vi "Invert Data.vi"(8 "error in (no error)":errorcluster, 9 "Multiplot Representation In":T1, 10 "Actual Transform In":T5, 11 "3D Plot.lvclass in":refnum<class "3D Plot.lvclass">) -> (0 "error out":errorcluster, 1 "Multiplot Representation In":T1, 2 "Actual Transform Out":T5, 3 "3D Plot.lvclass out":refnum<class "3D Plot.lvclass">)   [LabVIEW 2020, in "3D Plot.lvclass"]
uses:
  3D Plot.lvclass
  Actual Transform.ctl
  Range Clusters.ctl
  Multiplot Representation.ctl
  Plot Representation.ctl
  Mesh Data.ctl
  3D Plot.lvclass/3D Plot.ctl
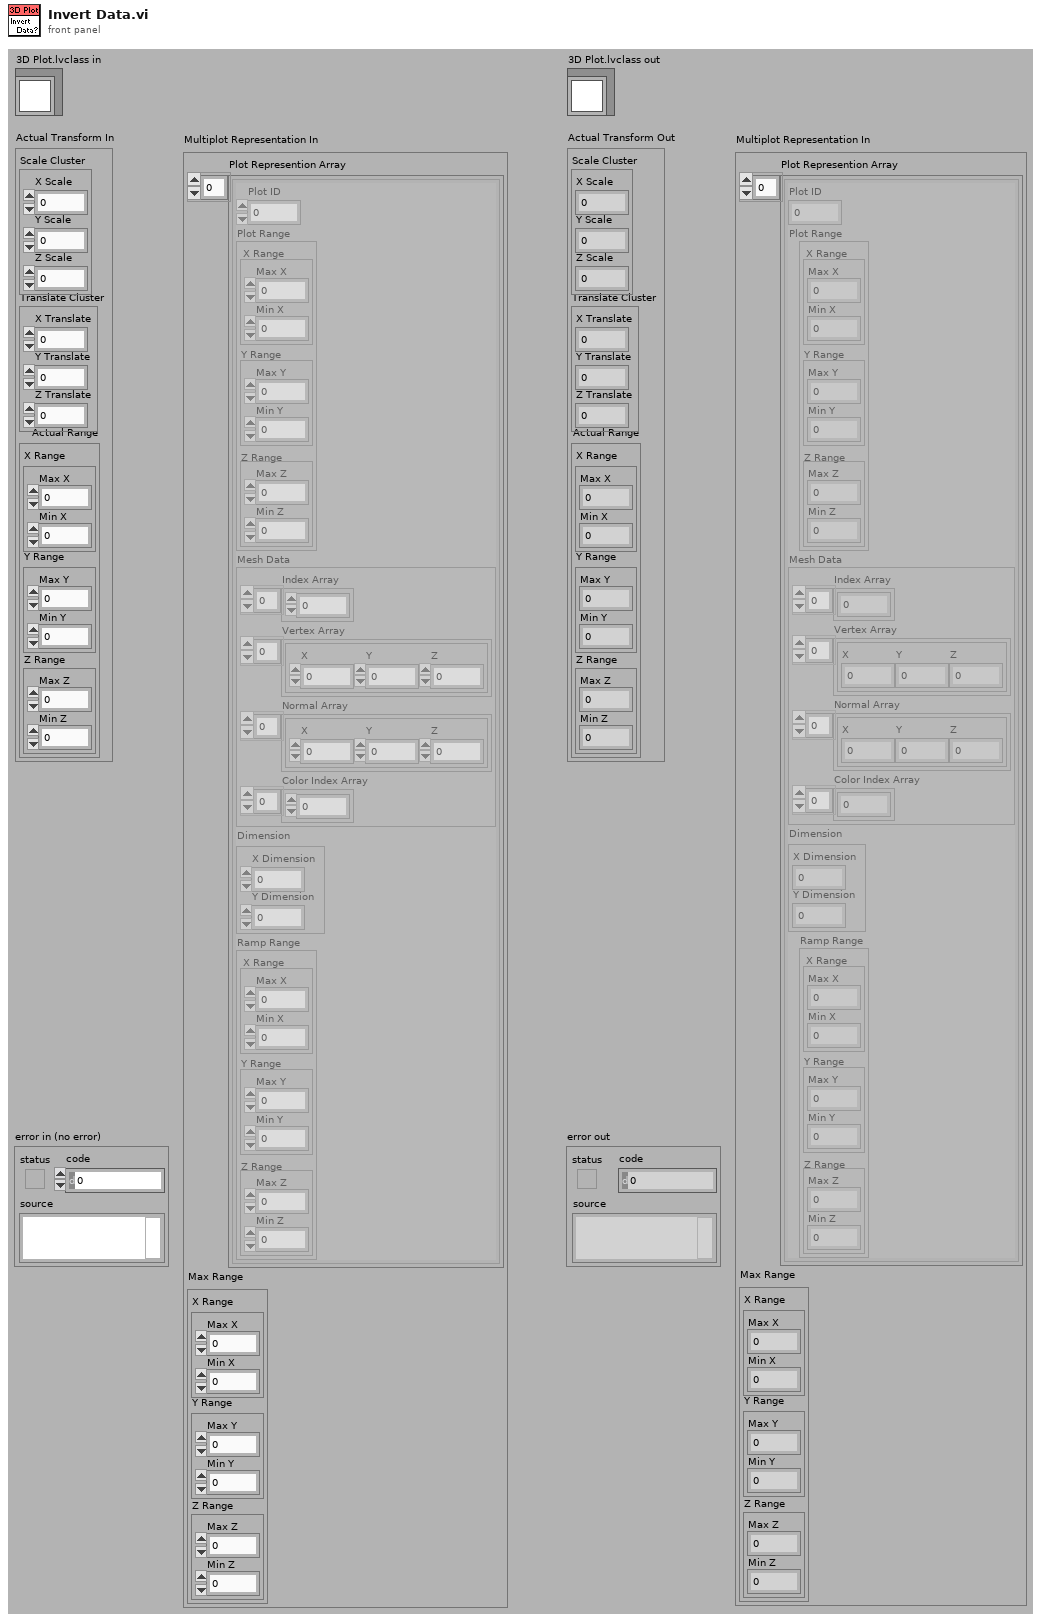
[diagram p1: front panel]
types:
  T1 = typedef "3D Plot.lvclass/Multiplot Representation.ctl" = cluster{"Plot Represention Array":T2[], "Max Range":T3}
  T2 = typedef "3D Plot.lvclass/Plot Representation.ctl" = cluster{"Plot ID":i32, "Plot Range":T3, "Mesh Data":T4, "Dimension":cluster{"X Dimension":i32, "Y Dimension":i32}, "Ramp Range":T3}
  T3 = typedef "3D Plot.lvclass/Range Clusters.ctl" = cluster{"X Range":cluster{"Max X":sgl, "Min X":sgl}, "Y Range":cluster{"Max Y":sgl, "Min Y":sgl}, "Z Range":cluster{"Max Z":sgl, "Min Z":sgl}}
  T4 = typedef "3D Plot.lvclass/Mesh Data.ctl" = cluster{"Index Array":u32[], "Vertex Array":cluster{"X":sgl, "Y":sgl, "Z":sgl}[], "Normal Array":cluster{"X":sgl, "Y":sgl, "Z":sgl}[], "Color Index Array":i32[]}
  T5 = typedef "3D Plot.lvclass/Actual Transform.ctl" = cluster{"Scale Cluster":cluster{"X Scale":sgl, "Y Scale":sgl, "Z Scale":sgl}, "Translate Cluster":cluster{"X Translate":sgl, "Y Translate":sgl, "Z Translate":sgl}, "Actual Range":T3}
  T6 = cluster{"Inverted X":bool, "Inverted Y":bool, "Inverted Z":bool}
  T7 = cluster{"Vertex":sgl, "Vertex":sgl, "Vertex":sgl}
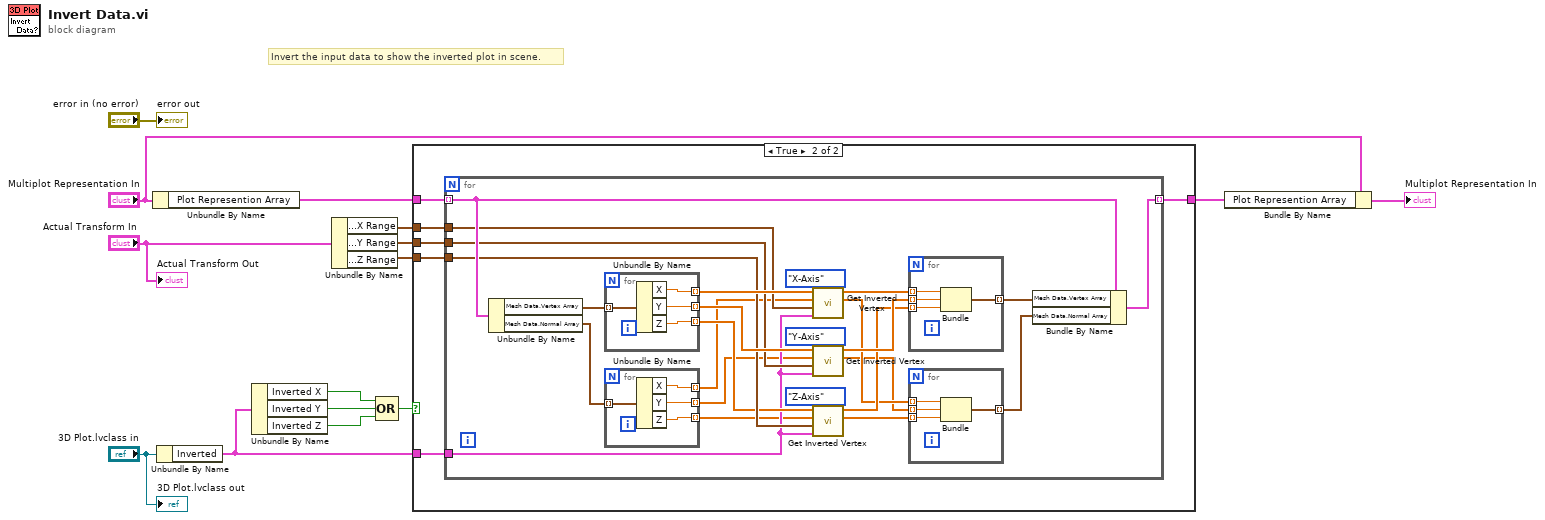
[diagram p0: block diagram]
diagram:
  # "Invert the input data to show the inverted plot in scene."
  n1 = Unbundle By Name("Multiplot Representation In") -> ("Plot Represention Array"=w3:T2[])
  n2 = Unbundle By Name("3D Plot.lvclass in") -> ("Inverted"=w1:T6)
  n3 = Unbundle By Name(w1) -> ("Inverted X"=w7:bool, "Inverted Y"=w6:bool, "Inverted Z"=w5:bool)
  n4 = Unbundle By Name("Actual Transform In") -> ("Actual Range.X Range"=w10:cluster{"Max X":sgl, "Min X":sgl}, "Actual Range.Y Range"=w9:cluster{"Max Y":sgl, "Min Y":sgl}, "Actual Range.Z Range"=w8:cluster{"Max Z":sgl, "Min Z":sgl})
  n5 = Compound Arithmetic op=OR(w7, w6, w5) -> (w4:bool)
  n6 = case shown="True" w4 {
    tunnel: w10 -> [_ w22]
    tunnel: w9 -> [_ w21]
    tunnel: w8 -> [_ w20]
    tunnel: w3 -> [w16 w19]
    tunnel: [w16 w18] -> w2
    tunnel: w1 -> [_ w17]
    frame False {
    }
    frame True {
      n7 = for {
        tunnel: w22 -> [w42]
        tunnel: w21 -> [w40]
        tunnel: w20 -> [w39]
        tunnel: w19 -> [w46] mode=indexing
        tunnel: [w47] -> w18 mode=indexing
        tunnel: w17 -> [w35]
        n8 = Unbundle By Name(w46) -> ("Mesh Data.Vertex Array"=w45:cluster{"X":sgl, "Y":sgl, "Z":sgl}[], "Mesh Data.Normal Array"=w30:cluster{"X":sgl, "Y":sgl, "Z":sgl}[])
        n9 = for {
          tunnel: w45 -> [w63] mode=indexing
          tunnel: [w62] -> w43 mode=indexing
          tunnel: [w61] -> w41 mode=indexing
          tunnel: [w60] -> w38 mode=indexing
          n10 = Unbundle By Name(w63) -> ("X"=w62:sgl, "Y"=w61:sgl, "Z"=w60:sgl)
        }
        n11 = for {
          tunnel: w30 -> [w55] mode=indexing
          tunnel: [w54] -> w29 mode=indexing
          tunnel: [w53] -> w28 mode=indexing
          tunnel: [w52] -> w27 mode=indexing
          n12 = Unbundle By Name(w55) -> ("X"=w54:sgl, "Y"=w53:sgl, "Z"=w52:sgl)
        }
        n13 = call "Get Inverted Vertex.vi"("Axis"=enum16{"X-Axis", "Y-Axis", "Z-Axis"}."X-Axis", "Inverted?"=w35, "Range In"=w42, "Normal Array In"=w29, "Vertex Array In"=w43) -> ("Normal Array Out"=w25:sgl[], "Vertex Array Out"=w31:sgl[])  [unwired: 5 out]
        n14 = call "Get Inverted Vertex.vi"("Axis"=enum16{"X-Axis", "Y-Axis", "Z-Axis"}."Y-Axis", "Inverted?"=w35, "Range In"=w40, "Normal Array In"=w28, "Vertex Array In"=w41) -> ("Normal Array Out"=w24:sgl[], "Vertex Array Out"=w37:sgl[])  [unwired: 5 out]
        n15 = call "Get Inverted Vertex.vi"("Axis"=enum16{"X-Axis", "Y-Axis", "Z-Axis"}."Z-Axis", "Inverted?"=w35, "Range In"=w39, "Normal Array In"=w27, "Vertex Array In"=w38) -> ("Normal Array Out"=w23:sgl[], "Vertex Array Out"=w36:sgl[])  [unwired: 5 out]
        n16 = for {
          tunnel: [w59] -> w44 mode=indexing
          tunnel: w31 -> [w58] mode=indexing
          tunnel: w37 -> [w57] mode=indexing
          tunnel: w36 -> [w56] mode=indexing
          n17 = Bundle("Vertex"=w58, "Vertex"=w57, "Vertex"=w56) -> (w59:T7)  [unwired: 1 out]
        }
        n18 = for {
          tunnel: [w51] -> w26 mode=indexing
          tunnel: w25 -> [w50] mode=indexing
          tunnel: w24 -> [w49] mode=indexing
          tunnel: w23 -> [w48] mode=indexing
          n19 = Bundle("Vertex"=w50, "Vertex"=w49, "Vertex"=w48) -> (w51:T7)  [unwired: 1 out]
        }
        n20 = Bundle By Name(cluster=w46, "Mesh Data.Vertex Array"=w44, "Mesh Data.Normal Array"=w26) -> (w47:T2)
      }
    }
  }
  n21 = Bundle By Name(cluster="Multiplot Representation In", "Plot Represention Array"=w2) -> (→"Multiplot Representation In":T1)
  "error out" <- "error in (no error)"
  "Actual Transform Out" <- "Actual Transform In"
  "3D Plot.lvclass out" <- "3D Plot.lvclass in"
